vi "Queue Nested.vi"(8 "Alias":string, 9 "Priority?":bool, 10 "Msg":refnum<class "Msg.lvclass">, 11 "Base Event Actor in":refnum<class "Base Event Actor.lvclass">) -> (3 "Base Event Actor out":refnum<class "Base Event Actor.lvclass">)   [LabVIEW 2021, in "jettl.lvlib" / "Base Event Actor.lvclass"]
uses:
  Base Event Actor.lvclass
  Msg/Msg/Msg.lvclass
  Base Event Actor.lvclass/Base Event Actor.ctl
  jettl.lvlib
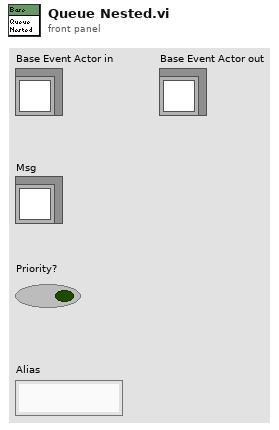
[diagram p1: front panel]
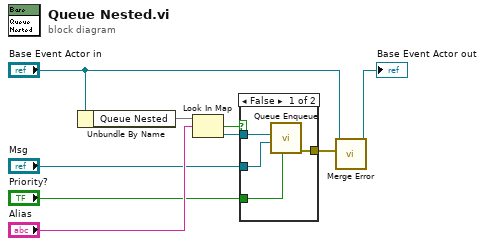
[diagram p0: block diagram]
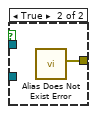
[diagram p2: hidden frame]
diagram:
  n1 = Unbundle By Name("Base Event Actor in") -> ("Queue Nested"=w8:map{string, refnum<data-value>})
  n2 = Look In Map(map=w8, key="Alias") -> (key not found?=w7:bool, value=w9:refnum<data-value>)  [unwired: 1 in]
  n3 = case shown="False" w7 {
    tunnel: [w13 w14] -> w6
    tunnel: "Priority?" -> [w12 _]
    tunnel: "Msg" -> [w11 _]
    tunnel: w9 -> [w10 _]
    frame False {
      n4 = call "Queue Enqueue.vi"("Priority?"=w12, "Msg"=w11, "Queue"=w10) -> ("error out"=w13:errorcluster)  [unwired: 8 in]
    }
    frame True {
      n5 = call "Alias Does Not Exist Error.vi"() -> ("Error"=w14:errorcluster)  [unwired: 11 in]
    }
  }
  n6 = call-dynamic "Merge Error.vi"("Error"=w6, "Base Event Actor in"="Base Event Actor in") -> ("Base Event Actor out"=→"Base Event Actor out":refnum<class "Base Event Actor.lvclass">)  [unwired: 9 in]
